vi "black box control.vi"(8 "dt":dbl, 9 "setpoint":dbl, 10 "process variable":dbl, 11 "sample control module in":T1 {"output range"."output low" format="%.2f"; "output range"."output high" format="%.2f"}) -> (2 "output high":dbl, 3 "sample control module out":T1 {"output range"."output low" format="%.2f"; "output range"."output high" format="%.2f"})   [LabVIEW 2013, in "user tag bus module.lvclass"]
uses:
  user tag bus module.lvclass
  control module.ctl
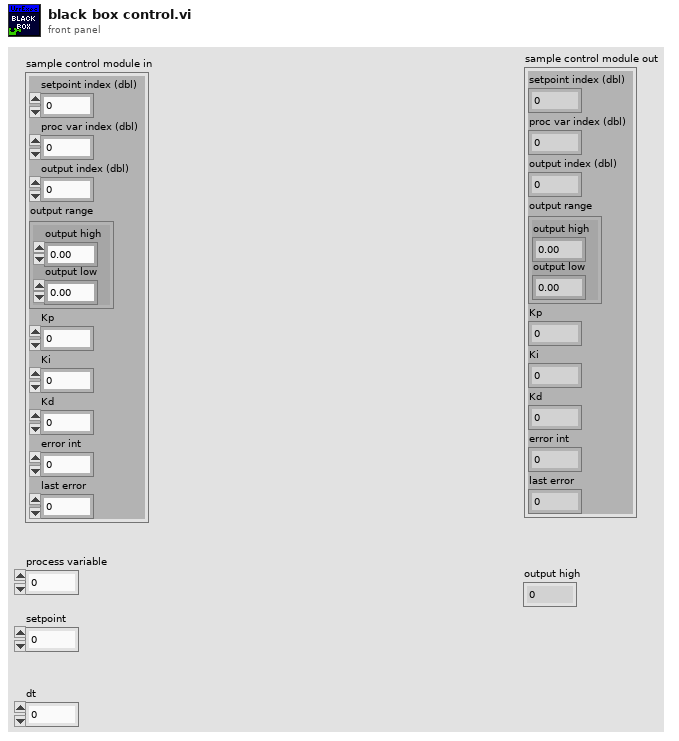
[diagram p1: front panel]
types:
  T1 = typedef "user tag bus module.lvclass/control module.ctl" = cluster{"setpoint index (dbl)":i32, "proc var index (dbl)":i32, "output index (dbl)":i32, "output range":cluster{"output high":dbl, "output low":dbl}, "Kp":dbl, "Ki":dbl, "Kd":dbl, "error int":dbl, "last error":dbl}
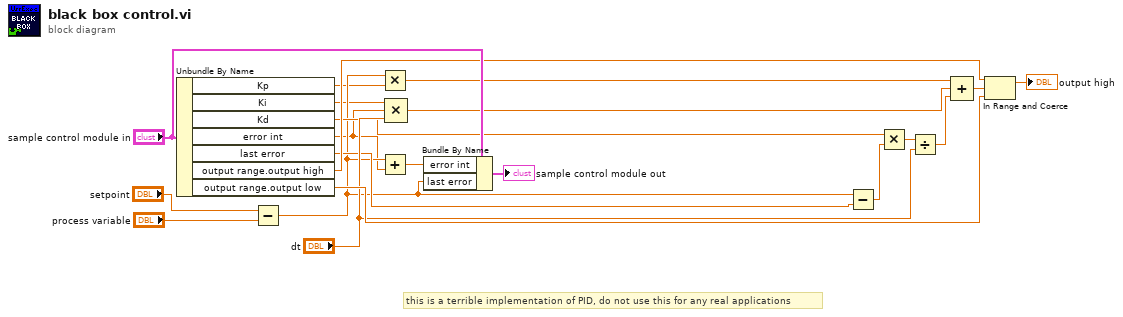
[diagram p0: block diagram]
diagram:
  # "this is a terrible implementation of PID, do not use this for any real applications"
  n1 = Unbundle By Name("sample control module in") -> ("Kp"=w4:dbl, "Ki"=w7:dbl, "Kd"=w12:dbl, "error int"=w6:dbl, "last error"=w10:dbl, "output range.output high"=w19:dbl, "output range.output low"=w20:dbl)
  n2 = Subtract(x="setpoint", y="process variable") -> (x-y=w9:dbl)
  n3 = Multiply(x=w9, y=w4) -> (x*y=w5:dbl)
  n4 = Add(x=w9, y=w6) -> (x+y=w16:dbl)
  n5 = Compound Arithmetic op=MULTIPLY(w7, w6, "dt") -> (w8:dbl)
  n6 = Bundle By Name(cluster="sample control module in", "error int"=w16, "last error"=w9) -> (→"sample control module out":T1)
  n7 = Subtract(x=w9, y=w10) -> (x-y=w11:dbl)
  n8 = Multiply(x=w12, y=w11) -> (x*y=w13:dbl)
  n9 = Divide(x=w13, y="dt") -> (x/y=w15:dbl)
  n10 = Compound Arithmetic op=ADD(w5, w8, w15) -> (w17:dbl)
  n11 = In Range and Coerce(upper limit=w19, x=w17, lower limit=w20) -> (coerced(x)=→"output high":dbl)  [unwired: 1 out]
